vi "relay_init.vi"(4 "VISA resource in":refnum<visa-resource-name>="COM12") -> (1 "relay session out":T1={"VISA resource out"="COM12", "error out"={"status"=FALSE, "code"=0, "source"=""}})   [LabVIEW 2010]
uses:
  <vilib>/Instr/_visa.llb/VISA Configure Serial Port (Instr).vi
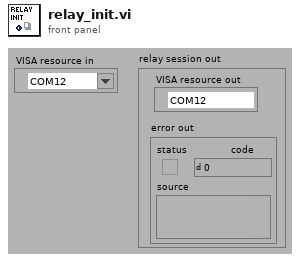
[diagram p1: front panel]
types:
  T1 = cluster{"VISA resource out":refnum<visa-resource-name>, "error out":errorcluster}
  T2 = cluster{"baud rate (9600)":u32, "data bits (8)":u16, "parity (0:none)":enum16{"None", "Odd", "Even", "Mark", "Space"}, "stop bits (10: 1 bit)":u16, "flow control (0:none)":u16, "timeout (10sec)":u32, "termination char\n(0xA = '\\n' = LF) ":u8, "Enable Termination\nChar (T)":bool}
  T3 = cluster{"VISA resource name out":refnum<visa-resource-name>, "error out":errorcluster}
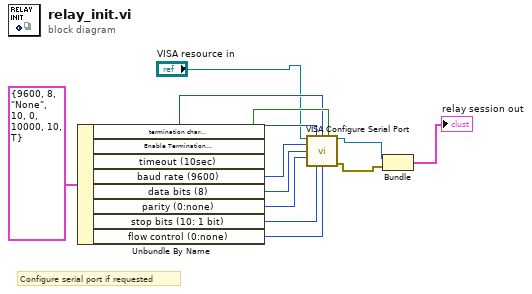
[diagram p0: block diagram]
diagram:
  # "Configure serial port if requested"
  n1 = Unbundle By Name(T2 {"baud rate (9600)"=9600, "data bits (8)"=8, "parity (0:none)"=enum."None", "stop bits (10: 1 bit)"=10, "flow control (0:none)"=0, "timeout (10sec)"=10000, "termination char\n(0xA = '\\n' = LF) "=10, "Enable Termination\nChar (T)"=TRUE} ("Port Configuration")) -> ("termination char\n(0xA = '\\n' = LF)"=w5:u8, "Enable Termination\nChar (T)"=w6:bool, "timeout (10sec)"=w7:u32, "baud rate (9600)"=w12:u32, "data bits (8)"=w11:u16, "parity (0:none)"=w10:enum16{"None", "Odd", "Even", "Mark", "Space"}, "stop bits (10: 1 bit)"=w9:u16, "flow control (0:none)"=w8:u16)
  n2 = call-poly "VISA Configure Serial Port"("VISA resource name"="VISA resource in", "timeout (10sec)"=w7, "termination char\n(0xA = '\\n' = LF)"=w5, "Enable Termination\nChar (T)"=w6, "baud rate (9600)"=w12, "data bits (8)"=w11, "parity (0:none)"=w10, "stop bits (10: 1 bit)"=w9, "flow control (0:none)"=w8) -> ("VISA resource name out"=w3:refnum<visa-resource-name>, "error out"=w2:errorcluster)  [unwired: 5 in]
  n3 = Bundle("VISA resource name out"=w3, "error out"=w2) -> (→"relay session out":T3)  [unwired: 1 in]
